vi "FGV_GuideTree.vi"(7 "Action":T1, 8 "error in":errorcluster caption="错误输入（无错误）", 11 "Tree*":refnum<vi>) -> (0 "error out":errorcluster caption="错误输出", 3 "Tree* out":refnum<vi>)   [LabVIEW 2016]
uses:
  FGV_GuideTree.ctl
  Modules/DAQ-Config/SubVIs/FGV_Cards.ctl
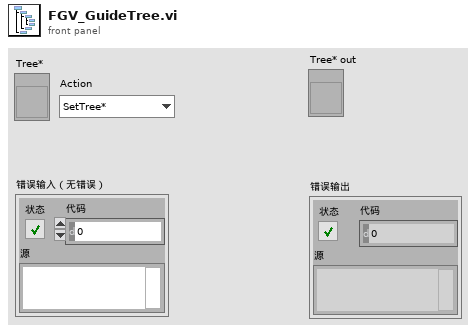
[diagram p1: front panel]
types:
  T1 = typedef "FGV_GuideTree.ctl" = enum16{"SetTree*", "GetTree*", "InitlizeTree", "AddCards"}
  T2 = cluster{"Left Cell String":string, "Child Text":string[], "Child Tag":string, "Item Indent":i32, "Child Only?":bool, "Glyph Index":i32}
  T3 = cluster{"父项标识符":string, "子项位置":i32, "子项标识符":string, "仅作为子项？":bool, "PicName":string, "左单元格字符串":string}
  T4 = typedef "FGV_Cards.ctl" = enum16{"Initlize", "Set_DAQCards", "Set_VCHCards", "Get_DAQCards", "Get_VCHCards", "Get_ALLUsing"}
  T5 = cluster{"TREE PNG":path, "User Guide":path, "DefaultSave":path, "BuildPath":path, "Image":path, "Modules":path, "Configuration":path, "License":path, "SplitFiles":path, "System.ini":path}
  T6 = typedef "PSCHN_Card Para.ctl" = cluster{"Module Type":string, "Module Name":string, "ModuSN":string, "ModuIP":string, "Used?":bool, "Connected":bool, "Timing*":cluster{"Sample Rate":dbl}, "Channels":T7[]}
  T7 = typedef "PSCHN_Channel Para.ctl" = cluster{"CHTag*":string, "Used?*":bool, "CHName":string, "Unit":string, "斜率":dbl, "截距":dbl}
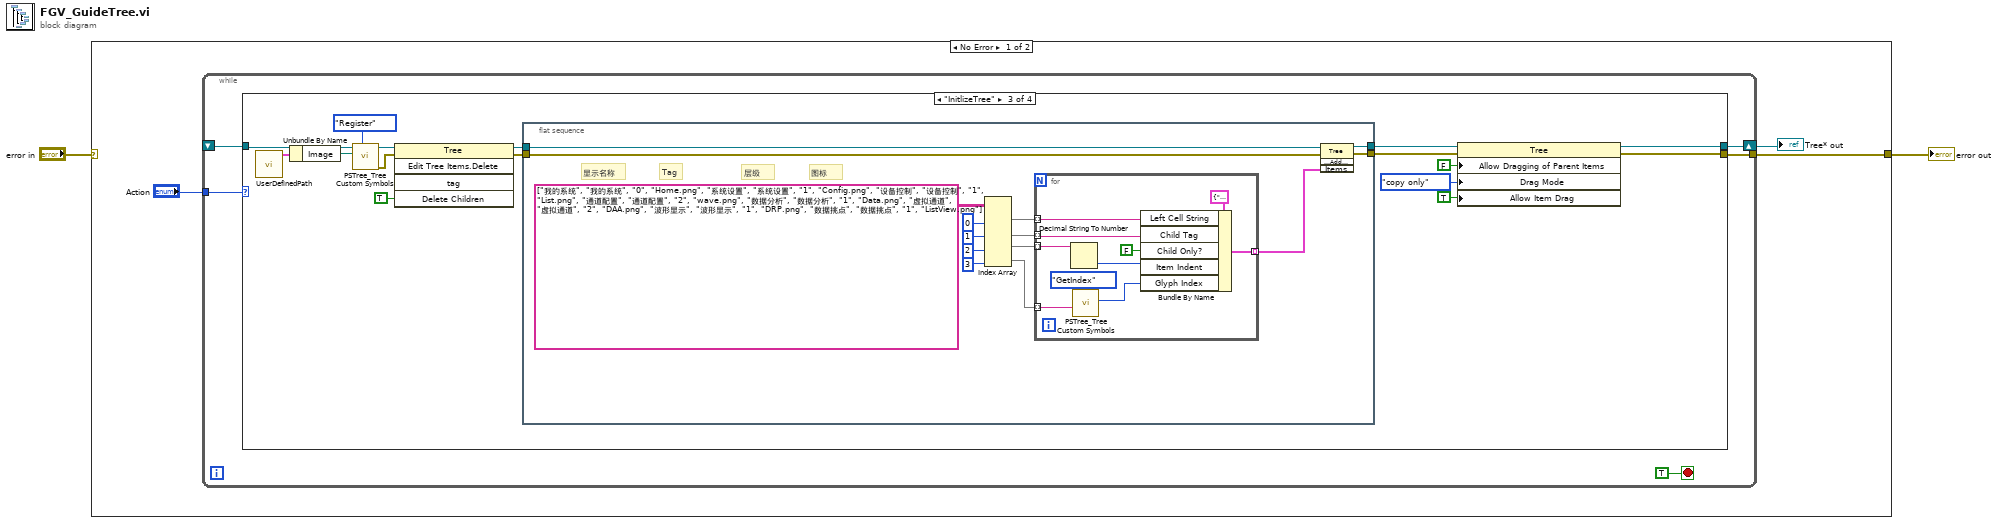
[diagram p0: block diagram]
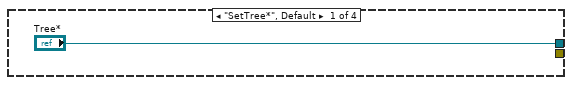
[diagram p2: hidden frame]
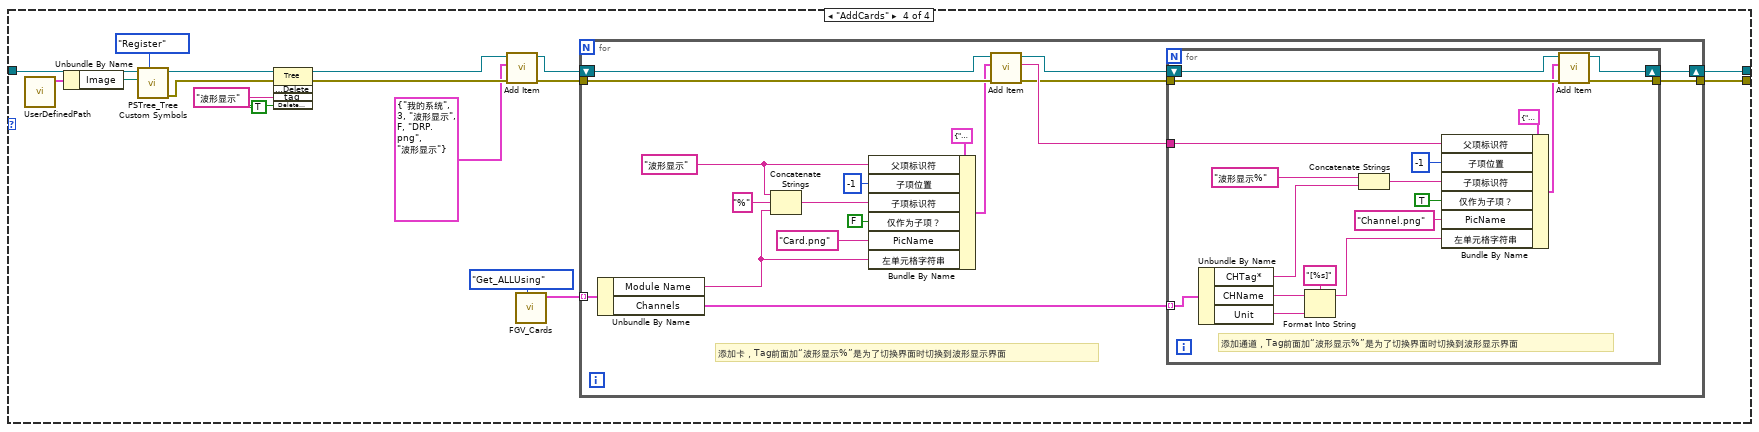
[diagram p4: hidden frame]
diagram:
  n1 = case shown="No Error" "error in" {
    selector: "error in" -> [_ w104]
    tunnel: [w3 w104] -> w2
    frame No Error {
      n2 = while {
        tunnel: "Action" -> [w9]
        shift-right: [w7] -> w4
        shift-left: _ -> [w8]
        tunnel: [w6] -> w3
        stop <- TRUE stop-if-true
        n3 = case shown="\"InitlizeTree\"" w9 {
          tunnel: w8 -> [_ w12 w22 w65]
          tunnel: ["Tree*" w12 w15 w62] -> w7
          tunnel: [_ _ w13 w53] -> w6
          frame "SetTree*", Default {
          }
          frame "GetTree*" {
          }
          frame "InitlizeTree" {
            n4 = call "UserDefinedPath.vi"() -> ("UserDefinedPath"=w21:T5)  [unwired: 11 in]
            n5 = Unbundle By Name(w21) -> ("Image"=w20:path)
            n6 = call "PSTree_Tree Custom Symbols.vi"("Operation"=enum16{"Register", "GetIndex"}."Register", "Files"=w20, "tree refnum"=w22) -> ("error out"=w26:errorcluster)  [unwired: 7 in, 1 out]
            n7 = invoke class="Tree" method="Edit Tree Items.Delete"(reference=w22, error in=w26, "Delete Children"=TRUE ("删除子项？")) -> (reference out=w24:refnum<vi>, error out=w25:errorcluster)  [unwired: 2 in, 3 out]
            n8 = flat-sequence {
              tunnel: w25 -> [w41]
              tunnel: w24 -> [w40]
              tunnel: [w29] -> w16
              tunnel: [w28] -> w14
              frame #0 {
                # "图标"
                # "层级"
                # "显示名称"
                # "Tag"
                n9 = Index Array(array=string[][] [["我的系统", "我的系统", "0", "Home.png"], ["系统设置", "系统设置", "1", "Config.png"], ["设备控制", "设备控制", "1", "List.png"], ["通道配置", "通道配置", "2", "wave.png"], ["数据分析", "数据分析", "1", "Data.png"], ["虚拟通道", "虚拟通道", "2", "DAA.png"], ["波形显示", "波形显示", "1", "DRP.png"], ["数据挑点", "数据挑点", "1", "ListView.png"]], index (col) #1=0 ("禁用的索引 (列)"), index (col) #2=1 ("索引 (列)"), index (col) #3=2 ("索引 (列)"), index (col) #4=3 ("索引 (列)")) -> (element #1=w37:string[], element #2=w33:string[], element #3=w30:string[], element #4=w31:string[])  [unwired: 4 in]
                n10 = for {
                  tunnel: [w50] -> w35 mode=indexing
                  tunnel: w37 -> [w47] mode=indexing
                  tunnel: w31 -> [w46] mode=indexing
                  tunnel: w33 -> [w44] mode=indexing
                  tunnel: w30 -> [w43] mode=indexing
                  n11 = Decimal String To Number(string=w43) -> (number=w45:i32)  [unwired: 2 in, 1 out]
                  n12 = call "PSTree_Tree Custom Symbols.vi"("Operation"=enum16{"Register", "GetIndex"}."GetIndex", "PicName"=w46) -> ("PicIndex"=w48:i32)  [unwired: 8 in, 1 out]
                  n13 = Bundle By Name(cluster=T2 {"Left Cell String"="", "Child Text"=[], "Child Tag"="", "Item Indent"=0, "Child Only?"=FALSE, "Glyph Index"=0} ("Item"), "Left Cell String"=w47, "Child Tag"=w44, "Child Only?"=FALSE, "Item Indent"=w45, "Glyph Index"=w48) -> (w50:T2)
                }
                n14 = invoke class="Tree" method="Edit Tree Items.Add Multiple Items to End"(reference=w40, error in=w41, "Items"=w35) -> (reference out=w29:refnum<vi>, error out=w28:errorcluster)  [unwired: 1 in, 2 out]
              }
            }
            n15 = property class="Tree"(reference=w16, error in=w14, "Allow Dragging of Parent Items"=FALSE ("拖曳/放置:允许拖曳父项"), "Drag Mode"=enum32{"copy or move", "copy only", "move only"}."copy only" ("拖曳/放置:拖曳模式"), "Allow Item Drag"=TRUE ("拖曳/放置:允许拖曳")) -> (reference out=w15:refnum<vi>, error out=w13:errorcluster)
          }
          frame "AddCards" {
            n16 = call "UserDefinedPath.vi"() -> ("UserDefinedPath"=w64:T5)  [unwired: 11 in]
            n17 = Unbundle By Name(w64) -> ("Image"=w63:path)
            n18 = call "PSTree_Tree Custom Symbols.vi"("Operation"=enum16{"Register", "GetIndex"}."Register", "Files"=w63, "tree refnum"=w65) -> ("error out"=w66:errorcluster)  [unwired: 7 in, 1 out]
            n19 = invoke class="Tree" method="Edit Tree Items.Delete"(reference=w65, error in=w66, "tag"="波形显示" ("父项标识符"), "Delete Children"=TRUE ("删除子项？")) -> (reference out=w57:refnum<vi>, error out=w56:errorcluster)  [unwired: 1 in, 3 out]
            n20 = call "Add Item.vi"("error in (no error)"=w56, "Info"=T3 {"父项标识符"="我的系统", "子项位置"=3, "子项标识符"="波形显示", "仅作为子项？"=FALSE, "PicName"="DRP.png", "左单元格字符串"="波形显示"}, "Tree"=w57) -> ("error out"=w54:errorcluster, "Tree out"=w55:refnum<vi>)  [unwired: 6 in, 1 out]
            n21 = call "FGV_Cards.vi"("Action"=FGV_Cards."Get_ALLUsing") -> ("Cards out"=w60:T6[])  [unwired: 9 in, 1 out]
            n22 = for {
              tunnel: w54 -> [w81]
              shift-right: [w83] -> w62
              shift-left: w55 -> [w80]
              tunnel: w60 -> [w85] mode=indexing
              tunnel: [w71] -> w53
              w77 = "波形显示" ("父项标识符")
              # "添加卡，Tag前面加“波形显示%”是为了切换界面时切换到波形显示界面"
              n23 = Unbundle By Name(w85) -> ("Module Name"=w69:string, "Channels"=w82:T7[])
              n24 = Concatenate Strings(w77, "%" ("字符串"), w69) -> (w76:string)
              n25 = Bundle By Name(cluster=T3 {"父项标识符"="波形显示%QX111", "子项位置"=-1, "子项标识符"="波形显示%2[MPa]", "仅作为子项？"=TRUE, "PicName"="Channel.png", "左单元格字符串"=""} ("Info"), "父项标识符"=w77, "子项位置"=-1, "子项标识符"=w76, "仅作为子项？"=FALSE, "PicName"="Card.png", "左单元格字符串"=w69) -> (w68:T3)
              n26 = call "Add Item.vi"("error in (no error)"=w81, "Info"=w68, "Tree"=w80) -> ("error out"=w72:errorcluster, "Tag"=w78:string, "Tree out"=w79:refnum<vi>)  [unwired: 6 in]
              n27 = for {
                shift-right: [w96] -> w83
                shift-left: w79 -> [w98]
                tunnel: w82 -> [w103] mode=indexing
                tunnel: w78 -> [w94]
                tunnel: w72 -> [w99]
                tunnel: [w95] -> w71
                # "添加通道，Tag前面加“波形显示%”是为了切换界面时切换到波形显示界面"
                n28 = Unbundle By Name(w103) -> ("CHTag*"=w86:string, "CHName"=w101:string, "Unit"=w100:string)
                n29 = Format Into String(format string="[%s]" ("格式字符串"), initial string=w101, w100) -> (resulting string=w88:string)  [unwired: 1 in, 1 out]
                n30 = Concatenate Strings("波形显示%" ("父项标识符"), w86) -> (w92:string)
                n31 = Bundle By Name(cluster=T3 {"父项标识符"="波形显示%QX111", "子项位置"=-1, "子项标识符"="波形显示%2[MPa]", "仅作为子项？"=TRUE, "PicName"="Channel.png", "左单元格字符串"=""} ("Info"), "父项标识符"=w94, "子项位置"=-1, "子项标识符"=w92, "仅作为子项？"=TRUE, "PicName"="Channel.png", "左单元格字符串"=w88) -> (w97:T3)
                n32 = call "Add Item.vi"("error in (no error)"=w99, "Info"=w97, "Tree"=w98) -> ("error out"=w95:errorcluster, "Tree out"=w96:refnum<vi>)  [unwired: 6 in, 1 out]
              }
            }
          }
        }
      }
      "Tree* out" <- w4
    }
    frame Error {
    }
  }
  "error out" <- w2
